vi "GUI.vi"() -> ()   [LabVIEW 2016]
uses:
  <vilib>/NI/Current Value Table/Type Defs/File Format.ctl
  <vilib>/NI/Current Value Table/Type Defs/Single Tag.ctl
  <vilib>/NI/Current Value Table/Type Defs/Data Types.ctl
  <vilib>/NI/Current Value Table/Type Defs/Tag Grouping set.ctl
  <vilib>/NI/Current Value Table/DataTypes/Boolean_Write.vi
  <vilib>/NI/Current Value Table/DataTypes/Boolean_Read.vi
  <vilib>/NI/Current Value Table/DataTypes/U16_Read.vi
  <vilib>/NI/Current Value Table/DataTypes/U16_Write.vi
  <vilib>/NI/Current Value Table/Type to Enum.vi
  <vilib>/NI/Current Value Table/DataTypes/Boolean_Type To Enum.vi
  <vilib>/NI/Current Value Table/DataTypes/U16_Type To Enum.vi
  MB_Master_Serial.lvclass
  C:/Users/PRANAV/Desktop/Modbus_Scada_Main/Modbus_Scada/MB_Master/MB_Master.lvclass
  MB_Master_TCP/MB_Master_TCP.lvclass
  <vilib>/NI/Current Value Table/FGVs/CVT Globals.vi
  <vilib>/NI/Current Value Table/FGVs/Tag Memory.vi
  <vilib>/NI/Current Value Table/Memory Block.vi
  <vilib>/NI/Current Value Table/DataTypes/Boolean_Memory Block.vi
  <vilib>/NI/Current Value Table/DataTypes/U16_Memory Block.vi
  MB_Master/MB_Master.lvclass
  <vilib>/NI/Current Value Table/Current Value Table.lvlib
  MB Master.lvlib
panel:
  in  "Type":enum16{"Serial", "TCP"}(ring) caption="Connection Type"
  out "Value_O2 3":u16
  out "Value_N2 3":u16
  out "Vel_Value 3":u16
  out "N2 Gas Pressure 1_Value 3":u16
  out "Temp_Min 4":u16
  out "Hum_Value  3":u16
  out "Value_O2 2":u16
  out "Value_N2 2":u16
  out "Vel_Value 2":u16
  out "N2 Gas Pressure 1_Value 2":u16
  out "Temp_Min 3":u16
  out "Hum_Value  2":u16
  out "Max_O2 2":u16
  out "Max_N2 2":u16
  out "Vel_Max 2":u16
  out "N2 Gas Pressure 1_Max 2":u16
  out "Temp_Max 2":u16
  out "Hum_Max 2":u16
  out "Min_O2 2":u16
  out "Min_N2 2":u16
  out "Vel_Min 2":u16
  out "N2 Gas Pressure 1_Min 2":u16
  out "Temp_Min 5":u16
  out "Hum_Min 2":u16
  out "Value_O2":u16
  out "Value_N2":u16
  out "Vel_Value":u16
  out "N2 Gas Pressure 1_Value":u16
  out "Temp_Min":u16
  out "Hum_Value":u16
  out "Spare AI-1_Value":u16
  out "Spare AI-2_Value":u16
  out "Max_O2":u16
  out "Max_N2":u16
  out "Vel_Max":u16
  out "N2 Gas Pressure 1_Max":u16
  out "Temp_Max":u16
  out "Hum_Max":u16
  out "Spare AI-1_Max":u16
  out "Spare AI-2_Max":u16
  out "Min_O2":u16
  out "Min_N2":u16
  out "Vel_Min":u16
  out "N2 Gas Pressure 1_Min":u16
  out "Temp_Min 2":u16
  out "Hum_Min":u16
  out "Spare AI-1_Min":u16
  out "Spare AI-2_Min":u16
  out "Value_8":bool
  out "Value_9":bool
  out "Value_10":bool
  out "Value_11":bool
  out "Value_12":bool
  out "Value_13":bool
  out "Value_14":bool
  out "Value_1":bool
  out "Value_2":bool
  out "Value_3":bool
  out "Value_4":bool
  out "Value_5":bool
  out "Value_6":bool
  out "Value_7":bool
  out "O.T. Entrance -Cap Proxy":bool
  out "Main Entrance E-stop PB":bool
  out "Doctors Entrance Door-2 Open Proxy FB":bool
  out "Main Entrance Door Open Inside PB":bool
  out "Main Entrance Door Open Proxy FB":bool
  out "O.T Entrance-Nose Mask Proxy":bool
  out "Doctors Entrance Door-1 Open PB":bool
  out "Doctors Entrance Door-1 Open Inside PB":bool
  out "Doctors Entrance Door-1 Open Proxy FB":bool
  out "Doctors Entrance-Nose Mask Proxy":bool
  out "Doctors Entrance-Cap Proxy":bool
  out "Doctors Entrance-Hand Sanitizer  Proxy":bool
  out "Doctors Entrance Door-2 Open Inside PB":bool
  out "Ist O.T.-Occupied Lamp Green":bool
  out "Ist O.T-AHU Start Coil":bool
  out "2nd O.T.:Scrubber Dispense Coil":bool
  out "2nd O.T.-Door Open Cmd":bool
  out "Spare DO-1":bool
  out "Spare DO-2":bool
  out "Spare DO-3":bool
  out "Spare DO-4":bool
  out "Spare DO-5":bool
  out "Spare DO-6":bool
  out "Doctor Entrance Door-1 Open Cmd":bool
  out "Doctor Entrance -Door-2 Open Cmd":bool
  out "Doctor Entrance -Hand Santizier Coil":bool
  out "Main Entrance-Door Open Cmd":bool
  out "OT Entrance-Door Open  Cmd":bool
  out "O.T Entrance-Hand Santiizier Coil":bool
  out "Ist O.T.- Door Open Cmd":bool
  out "Ist O.T-Occupied Lamp(Red)":bool
  out "Ist O.T-Inside Light":bool
  out "Ist O.T.-Scrubber Dispense Coil":bool
  out "error out":errorcluster
  in  "stop  5":bool
  in  "stop  4":bool
  in  "stop  3":bool
  in  "stop  2":bool
  in  "stop":bool
  # "DOORS &\n                    STATUS"
  # "Description"
  # "Status"
  # "Description"
  # "Status"
  # "Doctor Entrance Door-1 Open Cmd"
  # "Ist O.T.-Occupied Lamp Green"
  # "Doctor Entrance -Door-2 Open Cmd"
  # "Ist O.T-AHU Start Coil"
  # "Doctor Entrance -Hand Santizier Coil"
  # "2nd O.T.:Scrubber Dispense Coil"
  # "Main Entrance-Door Open Cmd"
  # "2nd O.T.-Door Open Cmd"
  # "OT Entrance-Door Open  Cmd"
  # "Spare DO-1"
  # "O.T Entrance-Hand Santiizier Coil"
  # "Spare DO-2"
  # "Ist O.T.- Door Open Cmd"
  # "Spare DO-3"
  # "Ist O.T-Occupied Lamp(Red)"
  # "Spare DO-4"
  # "Ist O.T-Inside Light"
  # "Spare DO-5"
  # "Ist O.T.-Scrubber Dispense Coil"
  # "Spare DO-6"
  # "DOORS FB AND SENSOR\n                                  STATUS"
  # "Description"
  # "Status"
  # "Description"
  # "Status"
  # "Doctors Entrance Door-1 Open PB"
  # "Doctors Entrance Door-2 Open Proxy FB"
  # "Doctors Entrance Door-1 Open Inside PB"
  # "Main Entrance E-stop PB"
  # "Doctors Entrance Door-1 Open Proxy FB"
  # "Main Entrance-Strecther Entry PB"
  # "Doctors Entrance-Nose Mask Proxy"
  # "Main Entrance Door Open Inside PB"
  # "Doctors Entrance-Cap Proxy"
  # "Main Entrance Door Open Proxy FB"
  # "Doctors Entrance-Hand Sanitizer  Proxy"
  # "O.T Entrance-Nose Mask Proxy"
  # "Doctors Entrance Door-2 Open Inside PB"
  # "O.T. Entrance -Cap Proxy"
  # "DOORS FB AND SENSOR\n                                  STATUS"
  # "Description"
  # "Status"
  # "Description"
  # "Status"
  # "OT Entrance-Hand Santizier Proxy"
  # "Spare DI-2"
  # "Spare DI-1"
  # "Ist O.T-AHU Run FB"
  # "OT Entrance-Door Inside Open PB"
  # "2nd O.T-Scrubber Proxy"
  # "OT Entrance-Door Open Proxy FB"
  # "2nd O.T-Door Inside Open PB"
  # "Ist O.T -Scrubber Proxy"
  # "2nd O.T-Door Open Proxy FB"
  # "Ist O.T-Door Inside Open PB"
  # "Ist O.T-E-Stop PB"
  # "Ist O.T-Door  Open Proxy FB"
  # "2nd O.T-E-Stop PB"
  # "O.T Parameters"
  # "Description"
  # "Min"
  # "Max"
  # "Value"
  # "Unit"
  # "O2 Gas Pressure"
  # "Bar"
  # "N2 Gas Pressure 1"
  # "Bar"
  # "Velocity"
  # "ft/m"
  # "N2 Gas Pressure 2"
  # "Bar"
  # "Room Temperature"
  # "Degree C"
  # "Relative Humidity"
  # "%"
  # "Spare AI 01"
  # "Spare AI 02"
  # "O.T Parameters S.P"
  # "Description"
  # "Very Low"
  # "Low"
  # "High"
  # "Very High"
  # "Unit"
  # "O2 Gas Pressure"
  # "Bar"
  # "N2 Gas Pressure 1"
  # "Bar"
  # "Velocity"
  # "ft/m"
  # "N2 Gas Pressure 2"
  # "Bar"
  # "Room Temperature"
  # "Degree C"
  # "Relative Humidity"
  # "%"
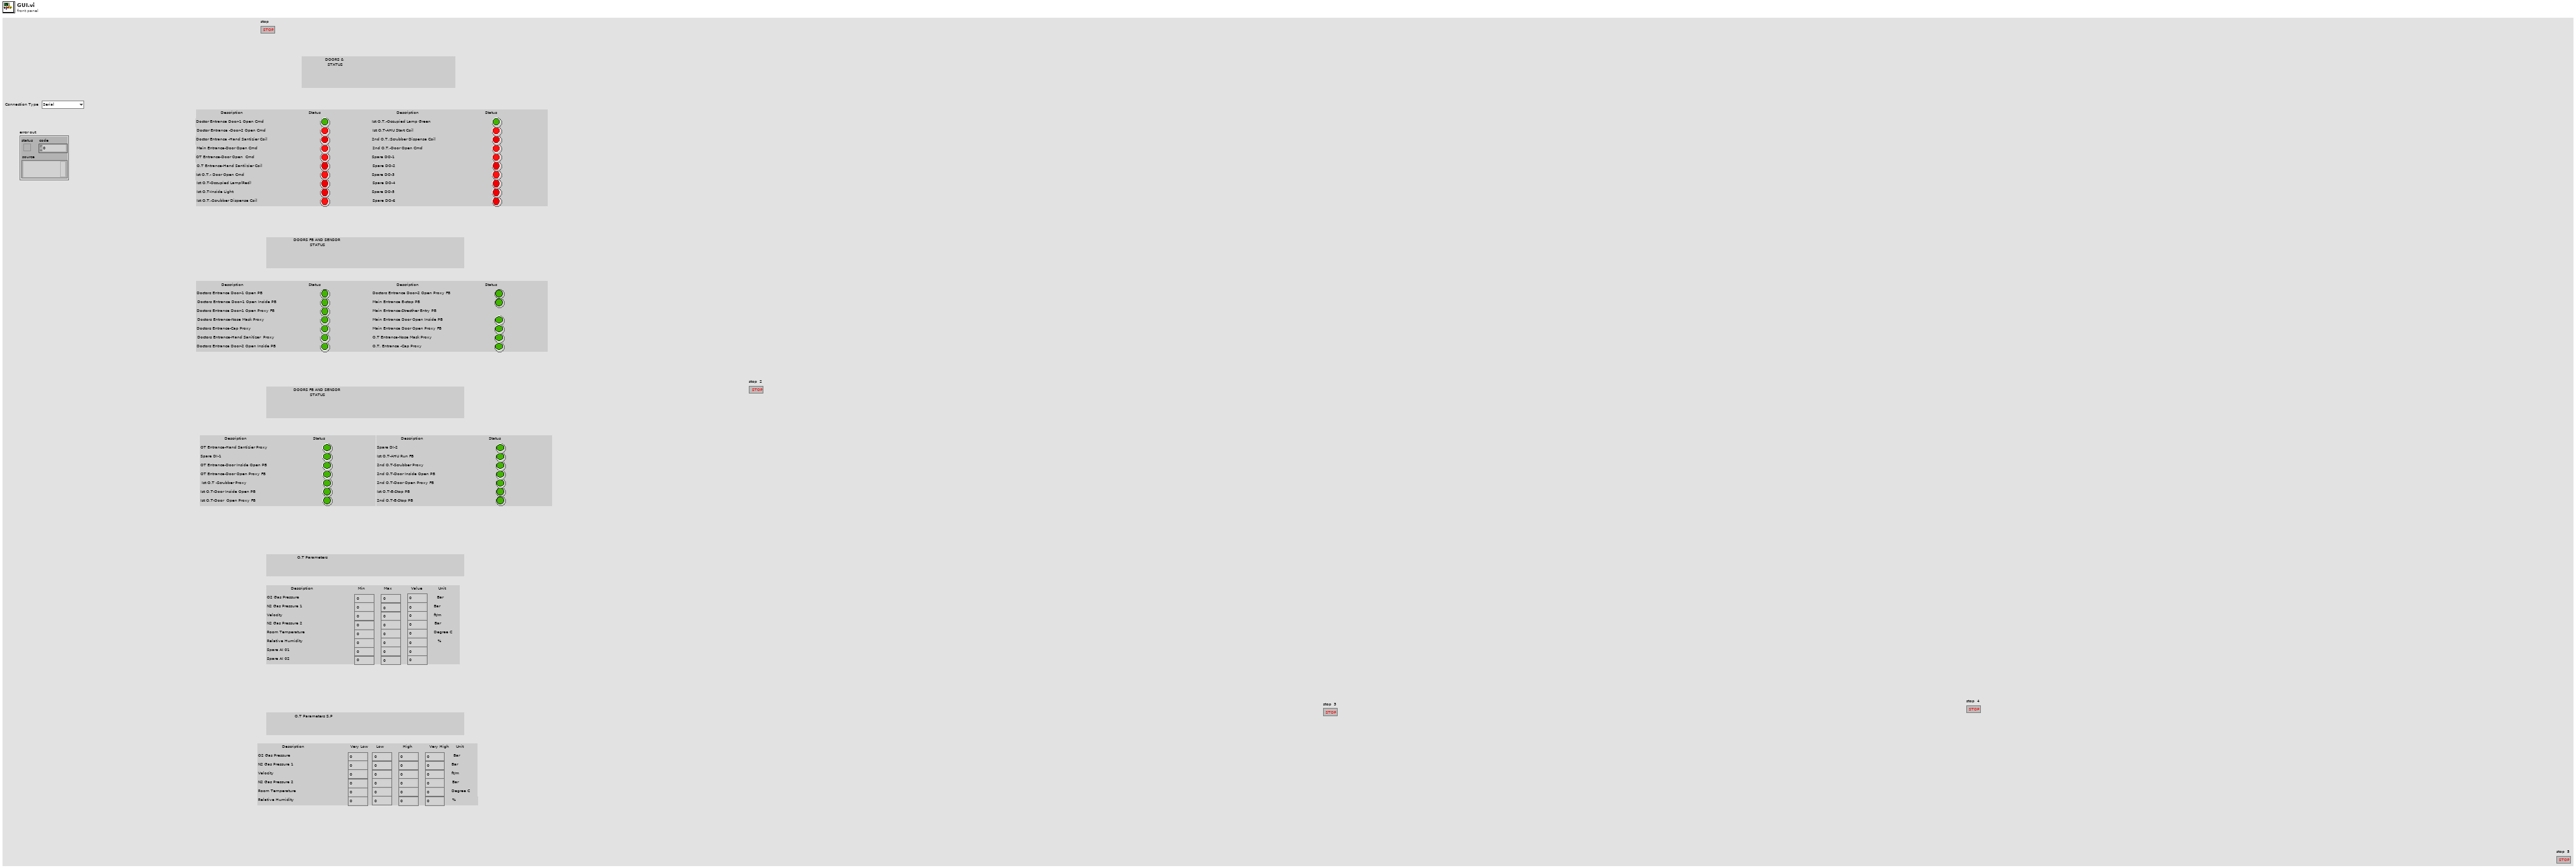
[diagram p1: front panel]
types:
  T1 = typedef "Current Value Table.lvlib/File Format.ctl" = cluster{"Tags":T2[], "Group Listings":T4[]}
  T2 = typedef "Current Value Table.lvlib/Single Tag.ctl" = cluster{"Data Type":T3, "Name":string, "Value":string, "Description":string}
  T3 = typedef "Current Value Table.lvlib/Data Types.ctl" = enum16{"Double", "Single", "I64", "I32", "I16", "I8", "U64", "U32", "U16", "U8", "String", "Boolean", "Array of U8", "Array of U16", "Array of U32", "Array of U64", "Array of I64", "Array of I32", "Array of I16", "Array of I8", "Array of Double", "Array of Single", "Array of Boolean", "Array of String"}
  T4 = typedef "Current Value Table.lvlib/Tag Grouping set.ctl" = cluster{"Group":string, "Tag Names":string[]}
  T5 = cluster{"baud rate (bps)":u32, "stop bits":u16, "parity":u16, "flow control":u16, "timeout":u32, "retries":i32}
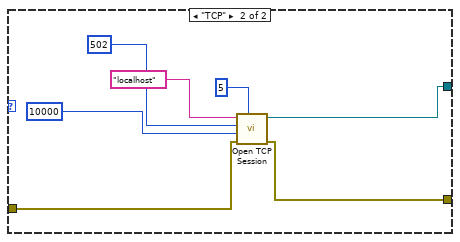
[diagram p2: hidden frame]
diagram:
  n1 = call <vilib>:"Create Tags.vi"("Clear Table? (F)"=FALSE, "CVT Tags to Create"=T1 {"Tags"=[{"Data Type"=enum."Boolean", "Name"="Doctor Entrance Door-1 Open Cmd", "Value"="", "Description"=""}, {"Data Type"=enum."Boolean", "Name"="Doctor Entrance -Door-2 Open Cmd", "Value"="", "Description"=""}, {"Data Type"=enum."Boolean", "Name"="Doctor Entrance -Hand Santizier Coil", "Value"="", "Description"=""}, {"Data Type"=enum."Boolean", "Name"="Main Entrance-Door Open Cmd", "Value"="", "Description"=""}, {"Data Type"=enum."Boolean", "Name"="OT Entrance-Door Open  Cmd", "Value"="", "Description"=""}, {"Data Type"=enum."Boolean", "Name"="O.T Entrance-Hand Santiizier Coil", "Value"="", "Description"=""}, {"Data Type"=enum."Boolean", "Name"="Ist O.T.- Door Open Cmd", "Value"="", "Description"=""}, {"Data Type"=enum."Boolean", "Name"="Ist O.T-Occupied Lamp(Red)", "Value"="", "Description"=""}, {"Data Type"=enum."Boolean", "Name"="Ist O.T-Inside Light", "Value"="", "Description"=""}, {"Data Type"=enum."Boolean", "Name"="Ist O.T.-Scrubber Dispense Coil", "Value"="", "Description"=""}, {"Data Type"=enum."Boolean", "Name"="Ist O.T.-Occupied Lamp Green", "Value"="", "Description"=""}, {"Data Type"=enum."Boolean", "Name"="Ist O.T-AHU Start Coil", "Value"="", "Description"=""}, {"Data Type"=enum."Boolean", "Name"="2nd O.T.:Scrubber Dispense Coil", "Value"="", "Description"=""}, {"Data Type"=enum."Boolean", "Name"="2nd O.T.-Door Open Cmd", "Value"="", "Description"=""}, {"Data Type"=enum."Boolean", "Name"="Spare DO-1", "Value"="", "Description"=""}, {"Data Type"=enum."Boolean", "Name"="Spare DO-2", "Value"="", "Description"=""}, {"Data Type"=enum."Boolean", "Name"="Spare DO-3", "Value"="", "Description"=""}, {"Data Type"=enum."Boolean", "Name"="Spare DO-4", "Value"="", "Description"=""}, {"Data Type"=enum."Boolean", "Name"="Spare DO-5", "Value"="", "Description"=""}, {"Data Type"=enum."Boolean", "Name"="Spare DO-6", "Value"="", "Description"=""}, {"Data Type"=enum."Boolean", "Name"="Doctors Entrance Door-1 Open PB ", "Value"="", "Description"=""}, {"Data Type"=enum."Boolean", "Name"="Doctors Entrance Door-1 Open Inside PB", "Value"="", "Description"=""}, {"Data Type"=enum."Boolean", "Name"="Doctors Entrance Door-1 Open Proxy FB", "Value"="", "Description"=""}, {"Data Type"=enum."Boolean", "Name"="Doctors Entrance-Nose Mask Proxy", "Value"="", "Description"=""}, {"Data Type"=enum."Boolean", "Name"="Doctors Entrance-Cap Proxy", "Value"="", "Description"=""}, {"Data Type"=enum."Boolean", "Name"="Doctors Entrance-Hand Sanitizer  Proxy", "Value"="", "Description"=""}, {"Data Type"=enum."Boolean", "Name"="Doctors Entrance Door-2 Open Inside PB", "Value"="", "Description"=""}, {"Data Type"=enum."Boolean", "Name"="Doctors Entrance Door-2 Open Proxy FB ", "Value"="", "Description"=""}, {"Data Type"=enum."Boolean", "Name"="Main Entrance E-stop PB", "Value"="", "Description"=""}, {"Data Type"=enum."Boolean", "Name"="Main Entrance-Strecther Entry PB ", "Value"="", "Description"=""}, {"Data Type"=enum."Boolean", "Name"="Main Entrance Door Open Inside PB", "Value"="", "Description"=""}, {"Data Type"=enum."Boolean", "Name"="Main Entrance Door Open Proxy FB", "Value"="", "Description"=""}, {"Data Type"=enum."Boolean", "Name"="O.T Entrance-Nose Mask Proxy ", "Value"="", "Description"=""}, {"Data Type"=enum."Boolean", "Name"="O.T. Entrance -Cap Proxy", "Value"="", "Description"=""}, {"Data Type"=enum."Boolean", "Name"="OT Entrance-Hand Santizier Proxy", "Value"="", "Description"=""}, {"Data Type"=enum."Boolean", "Name"="Spare DI-1", "Value"="", "Description"=""}, {"Data Type"=enum."Boolean", "Name"="OT Entrance-Door Inside Open PB ", "Value"="", "Description"=""}, {"Data Type"=enum."Boolean", "Name"="OT Entrance-Door Open Proxy FB ", "Value"="", "Description"=""}, {"Data Type"=enum."Boolean", "Name"="Ist O.T -Scrubber Proxy", "Value"="", "Description"=""}, {"Data Type"=enum."Boolean", "Name"="Ist O.T-Door Inside Open PB", "Value"="", "Description"=""}, {"Data Type"=enum."Boolean", "Name"="Ist O.T-Door  Open Proxy FB ", "Value"="", "Description"=""}, {"Data Type"=enum."Boolean", "Name"="Spare DI-2", "Value"="", "Description"=""}, {"Data Type"=enum."Boolean", "Name"="Ist O.T-AHU Run FB", "Value"="", "Description"=""}, {"Data Type"=enum."Boolean", "Name"="2nd O.T-Scrubber Proxy", "Value"="", "Description"=""}, {"Data Type"=enum."Boolean", "Name"="2nd O.T-Door Inside Open PB", "Value"="", "Description"=""}, {"Data Type"=enum."Boolean", "Name"="2nd O.T-Door Open Proxy FB ", "Value"="", "Description"=""}, {"Data Type"=enum."Boolean", "Name"="Ist O.T-E-Stop PB", "Value"="", "Description"=""}, {"Data Type"=enum."Boolean", "Name"="2nd O.T-E-Stop PB ", "Value"="", "Description"=""}, {"Data Type"=enum."U16", "Name"="O2 Gas Pressure_Min", "Value"="", "Description"=""}, {"Data Type"=enum."Double", "Name"="O2 Gas Pressure", "Value"="", "Description"=""}, {"Data Type"=enum."U16", "Name"="O2 Gas Pressure _Value", "Value"="", "Description"=""}, {"Data Type"=enum."U16", "Name"="O2 Gas Pressure_Max", "Value"="", "Description"=""}, {"Data Type"=enum."U16", "Name"="N2 Gas Pressure_Min", "Value"="", "Description"=""}, {"Data Type"=enum."U16", "Name"="N2 Gas Pressure_Max", "Value"="", "Description"=""}, {"Data Type"=enum."U16", "Name"="N2 Gas Pressure_Value", "Value"="", "Description"=""}, {"Data Type"=enum."U16", "Name"="Velocity_Min", "Value"="", "Description"=""}, {"Data Type"=enum."U16", "Name"="Velocity_Max", "Value"="", "Description"=""}, {"Data Type"=enum."U16", "Name"="Velocity_Value", "Value"="", "Description"=""}, {"Data Type"=enum."U16", "Name"="N2 Gas Pressure 1_Min", "Value"="", "Description"=""}, {"Data Type"=enum."U16", "Name"="N2 Gas Pressure 1 _Max", "Value"="", "Description"=""}, {"Data Type"=enum."U16", "Name"="N2 Gas Pressure 1_Value", "Value"="", "Description"=""}, {"Data Type"=enum."U16", "Name"="Temp_Min", "Value"="", "Description"=""}, {"Data Type"=enum."U16", "Name"="Temp_Max", "Value"="", "Description"=""}, {"Data Type"=enum."U16", "Name"="Temp_Value", "Value"="", "Description"=""}, {"Data Type"=enum."U16", "Name"="Hum_Min", "Value"="", "Description"=""}, {"Data Type"=enum."U16", "Name"="Hum_Max", "Value"="", "Description"=""}, {"Data Type"=enum."U16", "Name"="Hum_Value", "Value"="", "Description"=""}, {"Data Type"=enum."U16", "Name"="Spare AI-1_Min", "Value"="", "Description"=""}, {"Data Type"=enum."U16", "Name"="Spare AI-1_Max", "Value"="", "Description"=""}, {"Data Type"=enum."U16", "Name"="Spare AI-1_Value", "Value"="", "Description"=""}, {"Data Type"=enum."U16", "Name"="Spare AI-2_Min", "Value"="", "Description"=""}, {"Data Type"=enum."U16", "Name"="Spare AI-2_Max", "Value"="", "Description"=""}, {"Data Type"=enum."U16", "Name"="Spare AI-2_Value", "Value"="", "Description"=""}, {"Data Type"=enum."Boolean", "Name"="Value_1", "Value"="", "Description"=""}, {"Data Type"=enum."Boolean", "Name"="Value_2", "Value"="", "Description"=""}, {"Data Type"=enum."Boolean", "Name"="Value_3", "Value"="", "Description"=""}, {"Data Type"=enum."Boolean", "Name"="Value_4", "Value"="", "Description"=""}, {"Data Type"=enum."Boolean", "Name"="Value_5", "Value"="", "Description"=""}, {"Data Type"=enum."Boolean", "Name"="Value_6", "Value"="", "Description"=""}, {"Data Type"=enum."Boolean", "Name"="Value_7", "Value"="", "Description"=""}, {"Data Type"=enum."Boolean", "Name"="Value_8", "Value"="", "Description"=""}, {"Data Type"=enum."Boolean", "Name"="Value_9", "Value"="", "Description"=""}, {"Data Type"=enum."Boolean", "Name"="Value_10", "Value"="", "Description"=""}, {"Data Type"=enum."Boolean", "Name"="Value_11", "Value"="", "Description"=""}, {"Data Type"=enum."Boolean", "Name"="Value_12", "Value"="", "Description"=""}, {"Data Type"=enum."Boolean", "Name"="Value_13", "Value"="", "Description"=""}, {"Data Type"=enum."Boolean", "Name"="Value_14", "Value"="", "Description"=""}, {"Data Type"=enum."U16", "Name"="O2_L1", "Value"="", "Description"=""}, {"Data Type"=enum."U16", "Name"="O2_L2", "Value"="", "Description"=""}, {"Data Type"=enum."U16", "Name"="O2_H1", "Value"="", "Description"=""}, {"Data Type"=enum."U16", "Name"="O2_H2", "Value"="", "Description"=""}, {"Data Type"=enum."U16", "Name"="N21_L1", "Value"="", "Description"=""}, {"Data Type"=enum."U16", "Name"="N21_L2", "Value"="", "Description"=""}, {"Data Type"=enum."U16", "Name"="N21_H1", "Value"="", "Description"=""}, {"Data Type"=enum."U16", "Name"="N21_H2", "Value"="", "Description"=""}, {"Data Type"=enum."U16", "Name"="Vel_L1", "Value"="", "Description"=""}, {"Data Type"=enum."U16", "Name"="Vel_L2", "Value"="", "Description"=""}, {"Data Type"=enum."U16", "Name"="Vel_H1", "Value"="", "Description"=""}, {"Data Type"=enum."U16", "Name"="Vel_H2", "Value"="", "Description"=""}, {"Data Type"=enum."U16", "Name"="N22_L1", "Value"="", "Description"=""}, {"Data Type"=enum."U16", "Name"="N22_L2", "Value"="", "Description"=""}, {"Data Type"=enum."U16", "Name"="N22_H1", "Value"="", "Description"=""}, {"Data Type"=enum."U16", "Name"="N22_H2", "Value"="", "Description"=""}, {"Data Type"=enum."U16", "Name"="Temp_L1", "Value"="", "Description"=""}, {"Data Type"=enum."U16", "Name"="Temp_L2", "Value"="", "Description"=""}, {"Data Type"=enum."U16", "Name"="Temp_H1", "Value"="", "Description"=""}, {"Data Type"=enum."U16", "Name"="Temp_H2", "Value"="", "Description"=""}, {"Data Type"=enum."U16", "Name"="RH_L1", "Value"="", "Description"=""}, {"Data Type"=enum."U16", "Name"="RH_L2", "Value"="", "Description"=""}, {"Data Type"=enum."U16", "Name"="RH_H1", "Value"="", "Description"=""}, {"Data Type"=enum."U16", "Name"="RH_H2", "Value"="", "Description"=""}], "Group Listings"=[]}) -> ("error out"=w4:errorcluster)  [unwired: 9 in]
  n2 = case shown="\"Serial\", Default" "Type" {
    tunnel: [w14 w19] -> w2
    tunnel: [w13 w20] -> w3
    tunnel: w4 -> [w10 w17]
    frame "Serial", Default {
      n3 = call "Open Serial Session.vi"("Mode (RTU)"=enum16{"RTU", "ASCII"}."RTU", "Error in"=w10, "Slave ID"=u8 5, "Serial Config"=T5 {"baud rate (bps)"=19200, "stop bits"=10, "parity"=0, "flow control"=0, "timeout"=1000, "retries"=1}, "VISA Resource"=refnum<visa-resource-name> "COM9") -> ("Error out"=w14:errorcluster, "MB_Serial session"=w13:refnum<class "MB_Master_Serial.lvclass">)  [unwired: 5 in]
    }
    frame "TCP" {
      n4 = call "Open TCP Session.vi"("Slave ID (255)"=u8 5, "error in (no error)"=w17, "Timeout (10000)"=10000, "Port (502)"=u16 502, "IP Address"="localhost") -> ("error out"=w19:errorcluster, "MB_TCP session"=w20:refnum<class "MB_Master_TCP.lvclass">)  [unwired: 5 in]
    }
  }
  n5 = while {
    shift-right: [w39] -> w7
    shift-left: w3 -> [w40]
    shift-right: [w38] -> w6
    shift-left: w2 -> [w41]
    stop <- w24 stop-if-true
    n6 = flat-sequence {
      tunnel: w41 -> [w43]
      tunnel: w40 -> [w44]
      tunnel: [w168] -> w37
      tunnel: [w50] -> w36
      tunnel: [w46] -> w35
      tunnel: [w42] -> w34
      tunnel: w37 -> [_]
      tunnel: w36 -> [w177]
      tunnel: w35 -> [_]
      tunnel: w34 -> [w178]
      tunnel: [w247] -> w33
      tunnel: [w173] -> w32
      tunnel: [w172] -> w31
      tunnel: w33 -> [_]
      tunnel: w32 -> [w265]
      tunnel: w31 -> [w266]
      tunnel: [w400] -> w30
      tunnel: [w261] -> w29
      tunnel: [w262] -> w28
      tunnel: w30 -> [_]
      tunnel: w29 -> [w421]
      tunnel: w28 -> [w424]
      tunnel: [w420] -> w27
      tunnel: [w422] -> w26
      tunnel: [w504] -> w25
      tunnel: [w515] -> w39
      tunnel: [w516] -> w38
      tunnel: w27 -> [w517]
      tunnel: w26 -> [w513]
      tunnel: w25 -> [_]
      tunnel: [w636] -> w24
      frame #0 {
        w55 = "Spare DO-6" ("Tag Name")
        w62 = "Spare DO-5" ("Tag Name")
        w66 = "Spare DO-4" ("Tag Name")
        w70 = "Spare DO-3" ("Tag Name")
        w76 = "Spare DO-2" ("Tag Name")
        w49 = "Spare DO-1" ("Tag Name")
        w89 = "2nd O.T.-Door Open Cmd" ("Tag Name")
        w94 = "2nd O.T.:Scrubber Dispense Coil" ("Tag Name")
        w101 = "Ist O.T-AHU Start Coil" ("Tag Name")
        w104 = "Ist O.T.-Occupied Lamp Green" ("Tag Name")
        w113 = "Ist O.T.-Scrubber Dispense Coil" ("Tag Name")
        w117 = "Ist O.T-Inside Light" ("Tag Name")
        w125 = "Ist O.T-Occupied Lamp(Red)" ("Tag Name")
        w130 = "Ist O.T.- Door Open Cmd" ("Tag Name")
        w135 = "O.T Entrance-Hand Santiizier Coil" ("Tag Name")
        w153 = "OT Entrance-Door Open  Cmd" ("Tag Name")
        w156 = "Main Entrance-Door Open Cmd" ("Tag Name")
        w159 = "Doctor Entrance -Hand Santizier Coil" ("Tag Name")
        w165 = "Doctor Entrance -Door-2 Open Cmd" ("Tag Name")
        w171 = "Doctor Entrance Door-1 Open Cmd" ("Tag Name")
        n7 = call "Read Coils.vi"("error in (no error)"=w43, "quantity"=u16 22, "starting address"=u16 0, "MB session in"=w44) -> ("error out"=w45:errorcluster, "Coils"=w46:bool[], "MB session out"=w42:refnum<class "MB_Master.lvclass">)  [unwired: 5 in]
        n8 = Index Array(array=w46, index #1=0 ("index"), index #2=1 ("index"), index #3=2 ("index"), index #4=3 ("index"), index #5=4 ("index"), index #6=5 ("index"), index #7=6 ("index"), index #8=7 ("index"), index #9=8 ("index"), index #10=9 ("index"), index #11=10 ("index"), index #12=11 ("index"), index #13=12 ("index"), index #14=13 ("index"), index #15=14 ("index"), index #16=15 ("index"), index #17=16 ("index"), index #18=17 ("index"), index #19=18 ("index"), index #20=19 ("index")) -> (element #1=w148:bool, element #2=w146:bool, element #3=w144:bool, element #4=w142:bool, element #5=w140:bool, element #6=w138:bool, element #7=w132:bool, element #8=w126:bool, element #9=w120:bool, element #10=w114:bool, element #11=w108:bool, element #12=w102:bool, element #13=w96:bool, element #14=w90:bool, element #15=w83:bool, element #16=w78:bool, element #17=w73:bool, element #18=w67:bool, element #19=w63:bool, element #20=w54:bool)
        n9 = call-poly <vilib>:"Write.vi"("error in (no error)"=w45, "Value"=w148, "Tag Name"=w171) -> ("error out"=w164:errorcluster)  [unwired: 8 in]
        n10 = call-poly <vilib>:"Write.vi"("error in (no error)"=w164, "Value"=w146, "Tag Name"=w165) -> ("error out"=w161:errorcluster)  [unwired: 8 in]
        n11 = call-poly <vilib>:"Write.vi"("error in (no error)"=w161, "Value"=w144, "Tag Name"=w159) -> ("error out"=w157:errorcluster)  [unwired: 8 in]
        n12 = call-poly <vilib>:"Write.vi"("error in (no error)"=w157, "Value"=w142, "Tag Name"=w156) -> ("error out"=w150:errorcluster)  [unwired: 8 in]
        n13 = call-poly <vilib>:"Write.vi"("error in (no error)"=w150, "Value"=w140, "Tag Name"=w153) -> ("error out"=w137:errorcluster)  [unwired: 8 in]
        n14 = call-poly <vilib>:"Write.vi"("error in (no error)"=w137, "Value"=w138, "Tag Name"=w135) -> ("error out"=w131:errorcluster)  [unwired: 8 in]
        n15 = call-poly <vilib>:"Write.vi"("error in (no error)"=w131, "Value"=w132, "Tag Name"=w130) -> ("error out"=w124:errorcluster)  [unwired: 8 in]
        n16 = call-poly <vilib>:"Write.vi"("error in (no error)"=w124, "Value"=w126, "Tag Name"=w125) -> ("error out"=w119:errorcluster)  [unwired: 8 in]
        n17 = call-poly <vilib>:"Write.vi"("error in (no error)"=w119, "Value"=w120, "Tag Name"=w117) -> ("error out"=w112:errorcluster)  [unwired: 8 in]
        n18 = call-poly <vilib>:"Write.vi"("error in (no error)"=w112, "Value"=w114, "Tag Name"=w113) -> ("error out"=w105:errorcluster)  [unwired: 8 in]
        n19 = call-poly <vilib>:"Write.vi"("error in (no error)"=w105, "Value"=w108, "Tag Name"=w104) -> ("error out"=w100:errorcluster)  [unwired: 8 in]
        n20 = call-poly <vilib>:"Write.vi"("error in (no error)"=w100, "Value"=w102, "Tag Name"=w101) -> ("error out"=w95:errorcluster)  [unwired: 8 in]
        n21 = call-poly <vilib>:"Write.vi"("error in (no error)"=w95, "Value"=w96, "Tag Name"=w94) -> ("error out"=w88:errorcluster)  [unwired: 8 in]
        n22 = call-poly <vilib>:"Write.vi"("error in (no error)"=w88, "Value"=w90, "Tag Name"=w89) -> ("error out"=w85:errorcluster)  [unwired: 8 in]
        n23 = call-poly <vilib>:"Write.vi"("error in (no error)"=w85, "Value"=w83, "Tag Name"=w49) -> ("error out"=w80:errorcluster)  [unwired: 8 in]
        n24 = call-poly <vilib>:"Write.vi"("error in (no error)"=w80, "Value"=w78, "Tag Name"=w76) -> ("error out"=w72:errorcluster)  [unwired: 8 in]
        n25 = call-poly <vilib>:"Write.vi"("error in (no error)"=w72, "Value"=w73, "Tag Name"=w70) -> ("error out"=w60:errorcluster)  [unwired: 8 in]
        n26 = call-poly <vilib>:"Write.vi"("error in (no error)"=w60, "Value"=w67, "Tag Name"=w66) -> ("error out"=w61:errorcluster)  [unwired: 8 in]
        n27 = call-poly <vilib>:"Write.vi"("error in (no error)"=w61, "Value"=w63, "Tag Name"=w62) -> ("error out"=w53:errorcluster)  [unwired: 8 in]
        n28 = call-poly <vilib>:"Write.vi"("error in (no error)"=w53, "Value"=w54, "Tag Name"=w55) -> ()  [unwired: 8 in, 1 out]
        n29 = call-poly <vilib>:"Read.vi"("error in (no error)"=w164, "Tag Name"=w171) -> ("error out"=w163:errorcluster, "Value"=→"Doctor Entrance Door-1 Open Cmd":bool)  [unwired: 8 in]
        n30 = call-poly <vilib>:"Read.vi"("error in (no error)"=w163, "Tag Name"=w165) -> ("error out"=w160:errorcluster, "Value"=→"Doctor Entrance -Door-2 Open Cmd":bool)  [unwired: 8 in]
        n31 = call-poly <vilib>:"Read.vi"("error in (no error)"=w160, "Tag Name"=w159) -> ("error out"=w155:errorcluster, "Value"=→"Doctor Entrance -Hand Santizier Coil":bool)  [unwired: 8 in]
        n32 = Wait (ms)(milliseconds to wait=u32 500) -> ()  [unwired: 1 out]
        n33 = call-poly <vilib>:"Read.vi"("error in (no error)"=w155, "Tag Name"=w156) -> ("error out"=w152:errorcluster, "Value"=→"Main Entrance-Door Open Cmd":bool)  [unwired: 8 in]
        n34 = call-poly <vilib>:"Read.vi"("error in (no error)"=w152, "Tag Name"=w153) -> ("error out"=w136:errorcluster, "Value"=→"OT Entrance-Door Open  Cmd":bool)  [unwired: 8 in]
        n35 = call-poly <vilib>:"Read.vi"("error in (no error)"=w136, "Tag Name"=w135) -> ("error out"=w129:errorcluster, "Value"=→"O.T Entrance-Hand Santiizier Coil":bool)  [unwired: 8 in]
        n36 = call-poly <vilib>:"Read.vi"("error in (no error)"=w129, "Tag Name"=w130) -> ("error out"=w123:errorcluster, "Value"=→"Ist O.T.- Door Open Cmd":bool)  [unwired: 8 in]
        n37 = call-poly <vilib>:"Read.vi"("error in (no error)"=w123, "Tag Name"=w125) -> ("error out"=w118:errorcluster, "Value"=→"Ist O.T-Occupied Lamp(Red)":bool)  [unwired: 8 in]
        n38 = call-poly <vilib>:"Read.vi"("error in (no error)"=w118, "Tag Name"=w117) -> ("error out"=w111:errorcluster, "Value"=→"Ist O.T-Inside Light":bool)  [unwired: 8 in]
        n39 = call-poly <vilib>:"Read.vi"("error in (no error)"=w111, "Tag Name"=w113) -> ("error out"=w106:errorcluster, "Value"=→"Ist O.T.-Scrubber Dispense Coil":bool)  [unwired: 8 in]
        n40 = call-poly <vilib>:"Read.vi"("error in (no error)"=w106, "Tag Name"=w104) -> ("error out"=w99:errorcluster, "Value"=→"Ist O.T.-Occupied Lamp Green":bool)  [unwired: 8 in]
        n41 = call-poly <vilib>:"Read.vi"("error in (no error)"=w99, "Tag Name"=w101) -> ("error out"=w93:errorcluster, "Value"=→"Ist O.T-AHU Start Coil":bool)  [unwired: 8 in]
        n42 = call-poly <vilib>:"Read.vi"("error in (no error)"=w93, "Tag Name"=w94) -> ("error out"=w87:errorcluster, "Value"=→"2nd O.T.:Scrubber Dispense Coil":bool)  [unwired: 8 in]
        n43 = call-poly <vilib>:"Read.vi"("error in (no error)"=w87, "Tag Name"=w89) -> ("error out"=w82:errorcluster, "Value"=→"2nd O.T.-Door Open Cmd":bool)  [unwired: 8 in]
        n44 = call-poly <vilib>:"Read.vi"("error in (no error)"=w82, "Tag Name"=w49) -> ("error out"=w77:errorcluster, "Value"=→"Spare DO-1":bool)  [unwired: 8 in]
        n45 = call-poly <vilib>:"Read.vi"("error in (no error)"=w77, "Tag Name"=w76) -> ("error out"=w71:errorcluster, "Value"=→"Spare DO-2":bool)  [unwired: 8 in]
        n46 = call-poly <vilib>:"Read.vi"("error in (no error)"=w71, "Tag Name"=w70) -> ("error out"=w59:errorcluster, "Value"=→"Spare DO-3":bool)  [unwired: 8 in]
        n47 = call-poly <vilib>:"Read.vi"("error in (no error)"=w59, "Tag Name"=w66) -> ("error out"=w58:errorcluster, "Value"=→"Spare DO-4":bool)  [unwired: 8 in]
        n48 = call-poly <vilib>:"Read.vi"("error in (no error)"=w58, "Tag Name"=w62) -> ("error out"=w52:errorcluster, "Value"=→"Spare DO-5":bool)  [unwired: 8 in]
        n49 = call-poly <vilib>:"Read.vi"("error in (no error)"=w52, "Tag Name"=w55) -> ("error out"=w50:errorcluster, "Value"=→"Spare DO-6":bool)  [unwired: 8 in]
        n50 = Unbundle By Name(w50) -> ("status"=w169:bool)
        n51 = Or(x=w169, y="stop") -> (x .or. y?=w168:bool)
      }
      frame #1 {
        w185 = "O.T Entrance-Nose Mask Proxy " ("Tag Name")
        w190 = "Main Entrance Door Open Proxy FB" ("Tag Name")
        w195 = "Main Entrance Door Open Inside PB" ("Tag Name")
        w201 = "Doctors Entrance Door-2 Open Proxy FB " ("Tag Name")
        w207 = "Main Entrance E-stop PB" ("Tag Name")
        (unwired) FALSE ("Value")
        w213 = "O.T. Entrance -Cap Proxy" ("Tag Name")
        w221 = "Doctors Entrance Door-2 Open Inside PB" ("Tag Name")
        w224 = "Doctors Entrance-Hand Sanitizer  Proxy" ("Tag Name")
        w231 = "Doctors Entrance-Cap Proxy" ("Tag Name")
        w238 = "Doctors Entrance-Nose Mask Proxy" ("Tag Name")
        w244 = "Doctors Entrance Door-1 Open Proxy FB" ("Tag Name")
        w251 = "Doctors Entrance Door-1 Open Inside PB" ("Tag Name")
        w256 = "Doctors Entrance Door-1 Open PB " ("Tag Name")
        n52 = call "Read Discrete Inputs.vi"("error in (no error)"=w177, "quantity"=u16 16 ("Quantity"), "starting address"=u16 0 ("Starting Address"), "MB session in"=w178) -> ("error out"=w173:errorcluster, "Inputs"=w174:bool[], "MB session out"=w172:refnum<class "MB_Master.lvclass">)  [unwired: 5 in]
        n53 = Index Array(array=w174, index #1=0 ("index"), index #2=1 ("index"), index #3=2 ("index"), index #4=3 ("index"), index #5=4 ("index"), index #6=5 ("index"), index #7=6 ("index"), index #8=8 ("index"), index #9=9 ("index"), index #10=10 ("index"), index #11=11 ("index"), index #12=12 ("index"), index #13=13 ("index"), index #14=14 ("index")) -> (element #1=w259:bool, element #2=w252:bool, element #3=w245:bool, element #4=w239:bool, element #5=w233:bool, element #6=w225:bool, element #7=w219:bool, element #8=w215:bool, element #9=w209:bool, element #10=w202:bool, element #12=w196:bool, element #13=w192:bool, element #14=w186:bool)  [unwired: 1 out]
        n54 = call-poly <vilib>:"Write.vi"("Value"=w259, "Tag Name"=w256) -> ("error out"=w258:errorcluster)  [unwired: 9 in]
        n55 = call-poly <vilib>:"Write.vi"("error in (no error)"=w258, "Value"=w252, "Tag Name"=w251) -> ("error out"=w242:errorcluster)  [unwired: 8 in]
        n56 = call-poly <vilib>:"Write.vi"("error in (no error)"=w242, "Value"=w245, "Tag Name"=w244) -> ("error out"=w237:errorcluster)  [unwired: 8 in]
        n57 = call-poly <vilib>:"Write.vi"("error in (no error)"=w237, "Value"=w239, "Tag Name"=w238) -> ("error out"=w232:errorcluster)  [unwired: 8 in]
        n58 = call-poly <vilib>:"Write.vi"("error in (no error)"=w232, "Value"=w233, "Tag Name"=w231) -> ("error out"=w228:errorcluster)  [unwired: 8 in]
        n59 = call-poly <vilib>:"Write.vi"("error in (no error)"=w228, "Value"=w225, "Tag Name"=w224) -> ("error out"=w220:errorcluster)  [unwired: 8 in]
        n60 = call-poly <vilib>:"Write.vi"("error in (no error)"=w220, "Value"=w219, "Tag Name"=w221) -> ("error out"=w214:errorcluster)  [unwired: 8 in]
        n61 = call-poly <vilib>:"Write.vi"("error in (no error)"=w214, "Value"=w215, "Tag Name"=w213) -> ("error out"=w208:errorcluster)  [unwired: 8 in]
        n62 = call-poly <vilib>:"Write.vi"("error in (no error)"=w208, "Value"=w209, "Tag Name"=w207) -> ("error out"=w203:errorcluster)  [unwired: 8 in]
        n63 = call-poly <vilib>:"Write.vi"("error in (no error)"=w203, "Value"=w202, "Tag Name"=w201) -> ("error out"=w180:errorcluster)  [unwired: 8 in]
        n64 = call-poly <vilib>:"Write.vi"("error in (no error)"=w180, "Value"=w196, "Tag Name"=w195) -> ("error out"=w191:errorcluster)  [unwired: 8 in]
        n65 = call-poly <vilib>:"Write.vi"("error in (no error)"=w191, "Value"=w192, "Tag Name"=w190) -> ("error out"=w184:errorcluster)  [unwired: 8 in]
        n66 = call-poly <vilib>:"Write.vi"("error in (no error)"=w184, "Value"=w186, "Tag Name"=w185) -> ()  [unwired: 8 in, 1 out]
        n67 = call-poly <vilib>:"Read.vi"("error in (no error)"=w258, "Tag Name"=w256) -> ("error out"=w257:errorcluster, "Value"=→"Doctors Entrance Door-1 Open PB":bool)  [unwired: 8 in]
        n68 = call-poly <vilib>:"Read.vi"("error in (no error)"=w257, "Tag Name"=w251) -> ("error out"=w243:errorcluster, "Value"=→"Doctors Entrance Door-1 Open Inside PB":bool)  [unwired: 8 in]
        n69 = call-poly <vilib>:"Read.vi"("error in (no error)"=w243, "Tag Name"=w244) -> ("error out"=w236:errorcluster, "Value"=→"Doctors Entrance Door-1 Open Proxy FB":bool)  [unwired: 8 in]
        n70 = call-poly <vilib>:"Read.vi"("error in (no error)"=w236, "Tag Name"=w238) -> ("error out"=w230:errorcluster, "Value"=→"Doctors Entrance-Nose Mask Proxy":bool)  [unwired: 8 in]
        n71 = call-poly <vilib>:"Read.vi"("error in (no error)"=w230, "Tag Name"=w231) -> ("error out"=w227:errorcluster, "Value"=→"Doctors Entrance-Cap Proxy":bool)  [unwired: 8 in]
        n72 = call-poly <vilib>:"Read.vi"("error in (no error)"=w227, "Tag Name"=w224) -> ("error out"=w217:errorcluster, "Value"=→"Doctors Entrance-Hand Sanitizer  Proxy":bool)  [unwired: 8 in]
        n73 = call-poly <vilib>:"Read.vi"("error in (no error)"=w217, "Tag Name"=w221) -> ("error out"=w212:errorcluster, "Value"=→"Doctors Entrance Door-2 Open Inside PB":bool)  [unwired: 8 in]
        n74 = call-poly <vilib>:"Read.vi"("error in (no error)"=w212, "Tag Name"=w213) -> ("error out"=w206:errorcluster, "Value"=→"O.T. Entrance -Cap Proxy":bool)  [unwired: 8 in]
        n75 = call-poly <vilib>:"Read.vi"("error in (no error)"=w206, "Tag Name"=w207) -> ("error out"=w200:errorcluster, "Value"=→"Main Entrance E-stop PB":bool)  [unwired: 8 in]
        n76 = call-poly <vilib>:"Read.vi"("error in (no error)"=w200, "Tag Name"=w201) -> ("error out"=w179:errorcluster, "Value"=→"Doctors Entrance Door-2 Open Proxy FB":bool)  [unwired: 8 in]
        n77 = call-poly <vilib>:"Read.vi"("error in (no error)"=w179, "Tag Name"=w195) -> ("error out"=w189:errorcluster, "Value"=→"Main Entrance Door Open Inside PB":bool)  [unwired: 8 in]
        n78 = call-poly <vilib>:"Read.vi"("error in (no error)"=w189, "Tag Name"=w190) -> ("error out"=w183:errorcluster, "Value"=→"Main Entrance Door Open Proxy FB":bool)  [unwired: 8 in]
        n79 = call-poly <vilib>:"Read.vi"("error in (no error)"=w183, "Tag Name"=w185) -> ("error out"=w182:errorcluster, "Value"=→"O.T Entrance-Nose Mask Proxy":bool)  [unwired: 8 in]
        n80 = Unbundle By Name(w182) -> ("status"=w248:bool)
        n81 = Or(x=w248, y="stop  2") -> (x .or. y?=w247:bool)
      }
      frame #2 {
        w274 = "Spare AI-2_Min" ("Tag Name")
        w275 = "Spare AI-2_Value" ("Tag Name")
        w276 = "Spare AI-2_Max" ("Tag Name")
        w293 = "Spare AI-1_Value" ("Tag Name")
        w294 = "Spare AI-1_Max" ("Tag Name")
        w296 = "Spare AI-1_Min" ("Tag Name")
        w310 = "Hum_Value" ("Tag Name")
        w311 = "Hum_Max" ("Tag Name")
        w312 = "Hum_Min" ("Tag Name")
        w330 = "Temp_Value" ("Tag Name")
        w329 = "Temp_Max" ("Tag Name")
        w327 = "Temp_Min" ("Tag Name")
        w343 = "N2 Gas Pressure 1_Value" ("Tag Name")
        w348 = "N2 Gas Pressure 1 _Max" ("Tag Name")
        w349 = "N2 Gas Pressure 1_Min" ("Tag Name")
        w363 = "Velocity_Value" ("Tag Name")
        w365 = "Velocity_Max" ("Tag Name")
        w368 = "Velocity_Min" ("Tag Name")
        w383 = "N2 Gas Pressure_Value" ("Tag Name")
        w388 = "N2 Gas Pressure_Max" ("Tag Name")
        w392 = "N2 Gas Pressure_Min" ("Tag Name")
        w398 = "O2 Gas Pressure _Value" ("Tag Name")
        w399 = "O2 Gas Pressure_Max" ("Tag Name")
        w406 = "O2 Gas Pressure_Min" ("Tag Name")
        n82 = call "Read Input Registers.vi"("error in (no error)"=w265, "quantity"=u16 25 ("Starting Address"), "starting address"=u16 0 ("Starting Address"), "MB session in"=w266) -> ("error out"=w261:errorcluster, "Registers"=w260:u16[], "MB session out"=w262:refnum<class "MB_Master.lvclass">)  [unwired: 5 in]
        n83 = Index Array(array=w260, index #1=21 ("index"), index #2=22 ("index"), index #3=23 ("index")) -> (element #1=w279:u16, element #2=w278:u16, element #3=w277:u16)
        n84 = Index Array(array=w260, index #1=3 ("index"), index #2=4 ("index"), index #3=5 ("index")) -> (element #1=w394:u16, element #2=w389:u16, element #3=w381:u16)
        n85 = Index Array(array=w260, index #1=18 ("index"), index #2=19 ("index"), index #3=20 ("index")) -> (element #1=w299:u16, element #2=w298:u16, element #3=w297:u16)
        n86 = Index Array(array=w260, index #1=6 ("index"), index #2=7 ("index"), index #3=8 ("index")) -> (element #1=w373:u16, element #2=w372:u16, element #3=w371:u16)
        n87 = Index Array(array=w260, index #1=9 ("index"), index #2=10 ("index"), index #3=11 ("index")) -> (element #1=w356:u16, element #2=w355:u16, element #3=w354:u16)
        n88 = Index Array(array=w260, index #1=12 ("index"), index #2=13 ("index"), index #3=14 ("index")) -> (element #1=w338:u16, element #2=w337:u16, element #3=w336:u16)
        n89 = Index Array(array=w260, index #1=0 ("index"), index #2=1 ("index"), index #3=2 ("index")) -> (element #1=w416:u16, element #2=w414:u16, element #3=w408:u16)
        n90 = Index Array(array=w260, index #1=15 ("index"), index #2=16 ("index"), index #3=17 ("index")) -> (element #1=w315:u16, element #2=w314:u16, element #3=w313:u16)
        n91 = call-poly <vilib>:"Write.vi"("error in (no error)"=w261, "Value"=w416, "Tag Name"=w406) -> ("error out"=w413:errorcluster)  [unwired: 8 in]
        n92 = call-poly <vilib>:"Read.vi"("error in (no error)"=w413, "Default"=u16 0, "Tag Name"=w406) -> ("error out"=w412:errorcluster, "Value"=→"Min_O2":u16)  [unwired: 7 in]
        n93 = call-poly <vilib>:"Read.vi"("Default"=u16 0, "Tag Name"=w392) -> ("error out"=w386:errorcluster, "Value"=→"Min_N2":u16)  [unwired: 8 in]
        n94 = call-poly <vilib>:"Write.vi"("error in (no error)"=w413, "Value"=w414, "Tag Name"=w399) -> ("error out"=w407:errorcluster)  [unwired: 8 in]
        n95 = call-poly <vilib>:"Read.vi"("error in (no error)"=w412, "Default"=u16 0, "Tag Name"=w399) -> ("error out"=w404:errorcluster, "Value"=→"Max_O2":u16)  [unwired: 7 in]
        n96 = call-poly <vilib>:"Read.vi"("Tag Name"=w329) -> ("error out"=w331:errorcluster, "Value"=→"Temp_Max":u16)  [unwired: 9 in]
        n97 = call-poly <vilib>:"Read.vi"("error in (no error)"=w386, "Default"=u16 0, "Tag Name"=w388) -> ("error out"=w379:errorcluster, "Value"=→"Max_N2":u16)  [unwired: 7 in]
        n98 = call-poly <vilib>:"Write.vi"("error in (no error)"=w407, "Value"=w408, "Tag Name"=w398) -> ()  [unwired: 8 in, 1 out]
        n99 = call-poly <vilib>:"Read.vi"("error in (no error)"=w331, "Tag Name"=w330) -> ("error out"=w308:errorcluster, "Value"=→"Temp_Min 2":u16)  [unwired: 8 in]
        n100 = call-poly <vilib>:"Read.vi"("error in (no error)"=w308, "Tag Name"=w312) -> ("error out"=w307:errorcluster, "Value"=→"Hum_Min":u16)  [unwired: 8 in]
        n101 = call-poly <vilib>:"Read.vi"("error in (no error)"=w307, "Tag Name"=w311) -> ("error out"=w318:errorcluster, "Value"=→"Hum_Max":u16)  [unwired: 8 in]
        n102 = call-poly <vilib>:"Read.vi"("error in (no error)"=w318, "Tag Name"=w310) -> ("error out"=w280:errorcluster, "Value"=→"Hum_Value":u16)  [unwired: 8 in]
        n103 = call-poly <vilib>:"Read.vi"("error in (no error)"=w280, "Default"=u16 0, "Tag Name"=w296) -> ("error out"=w303:errorcluster, "Value"=→"Spare AI-1_Min":u16)  [unwired: 7 in]
        n104 = call-poly <vilib>:"Read.vi"("error in (no error)"=w303, "Default"=u16 0, "Tag Name"=w294) -> ("error out"=w304:errorcluster, "Value"=→"Spare AI-1_Max":u16)  [unwired: 7 in]
        n105 = call-poly <vilib>:"Read.vi"("error in (no error)"=w304, "Default"=u16 0, "Tag Name"=w293) -> ("error out"=w272:errorcluster, "Value"=→"Spare AI-1_Value":u16)  [unwired: 7 in]
        n106 = call-poly <vilib>:"Read.vi"("error in (no error)"=w272, "Tag Name"=w274) -> ("error out"=w281:errorcluster, "Value"=→"Spare AI-2_Min":u16)  [unwired: 8 in]
        n107 = call-poly <vilib>:"Read.vi"("error in (no error)"=w281, "Tag Name"=w276) -> ("error out"=w282:errorcluster, "Value"=→"Spare AI-2_Max":u16)  [unwired: 8 in]
        n108 = call-poly <vilib>:"Read.vi"("error in (no error)"=w282, "Tag Name"=w275) -> ("error out"=w271:errorcluster, "Value"=→"Spare AI-2_Value":u16)  [unwired: 8 in]
        n109 = call-poly <vilib>:"Read.vi"("error in (no error)"=w379, "Default"=u16 0, "Tag Name"=w383) -> ("error out"=w367:errorcluster, "Value"=→"Value_N2":u16)  [unwired: 7 in]
        n110 = call-poly <vilib>:"Read.vi"("error in (no error)"=w367, "Tag Name"=w368) -> ("error out"=w366:errorcluster, "Value"=→"Vel_Min":u16)  [unwired: 8 in]
        n111 = call-poly <vilib>:"Read.vi"("error in (no error)"=w366, "Tag Name"=w365) -> ("error out"=w364:errorcluster, "Value"=→"Vel_Max":u16)  [unwired: 8 in]
        n112 = call-poly <vilib>:"Read.vi"("error in (no error)"=w364, "Tag Name"=w363) -> ("error out"=w350:errorcluster, "Value"=→"Vel_Value":u16)  [unwired: 8 in]
        n113 = call-poly <vilib>:"Read.vi"("error in (no error)"=w350, "Tag Name"=w349) -> ("error out"=w347:errorcluster, "Value"=→"N2 Gas Pressure 1_Min":u16)  [unwired: 8 in]
        n114 = call-poly <vilib>:"Read.vi"("error in (no error)"=w347, "Tag Name"=w348) -> ("error out"=w344:errorcluster, "Value"=→"N2 Gas Pressure 1_Max":u16)  [unwired: 8 in]
        n115 = call-poly <vilib>:"Read.vi"("error in (no error)"=w344, "Tag Name"=w343) -> ("error out"=w328:errorcluster, "Value"=→"N2 Gas Pressure 1_Value":u16)  [unwired: 8 in]
        n116 = call-poly <vilib>:"Read.vi"("error in (no error)"=w328, "Tag Name"=w327) -> ("Value"=→"Temp_Min":u16)  [unwired: 8 in, 1 out]
        n117 = call-poly <vilib>:"Read.vi"("error in (no error)"=w404, "Default"=u16 0, "Tag Name"=w398) -> ("error out"=w393:errorcluster, "Value"=→"Value_O2":u16)  [unwired: 7 in]
        n118 = call-poly <vilib>:"Write.vi"("error in (no error)"=w393, "Value"=w394, "Tag Name"=w392) -> ("error out"=w387:errorcluster)  [unwired: 8 in]
        n119 = call-poly <vilib>:"Write.vi"("error in (no error)"=w387, "Value"=w389, "Tag Name"=w388) -> ("error out"=w384:errorcluster)  [unwired: 8 in]
        n120 = call-poly <vilib>:"Write.vi"("error in (no error)"=w384, "Value"=w381, "Tag Name"=w383) -> ("error out"=w374:errorcluster)  [unwired: 8 in]
        n121 = call-poly <vilib>:"Write.vi"("error in (no error)"=w374, "Value"=w373, "Tag Name"=w368) -> ("error out"=w370:errorcluster)  [unwired: 8 in]
        n122 = call-poly <vilib>:"Write.vi"("error in (no error)"=w370, "Value"=w372, "Tag Name"=w365) -> ("error out"=w369:errorcluster)  [unwired: 8 in]
        n123 = call-poly <vilib>:"Write.vi"("error in (no error)"=w369, "Value"=w371, "Tag Name"=w363) -> ("error out"=w353:errorcluster)  [unwired: 8 in]
        n124 = call-poly <vilib>:"Write.vi"("error in (no error)"=w353, "Value"=w356, "Tag Name"=w349) -> ("error out"=w352:errorcluster)  [unwired: 8 in]
        n125 = call-poly <vilib>:"Write.vi"("error in (no error)"=w352, "Value"=w355, "Tag Name"=w348) -> ("error out"=w351:errorcluster)  [unwired: 8 in]
        n126 = call-poly <vilib>:"Write.vi"("error in (no error)"=w351, "Value"=w354, "Tag Name"=w343) -> ("error out"=w335:errorcluster)  [unwired: 8 in]
        n127 = call-poly <vilib>:"Write.vi"("error in (no error)"=w335, "Value"=w338, "Tag Name"=w327) -> ("error out"=w334:errorcluster)  [unwired: 8 in]
        n128 = call-poly <vilib>:"Write.vi"("error in (no error)"=w334, "Value"=w337, "Tag Name"=w329) -> ("error out"=w333:errorcluster)  [unwired: 8 in]
        n129 = call-poly <vilib>:"Write.vi"("error in (no error)"=w333, "Value"=w336, "Tag Name"=w330) -> ("error out"=w309:errorcluster)  [unwired: 8 in]
        n130 = call-poly <vilib>:"Write.vi"("error in (no error)"=w309, "Value"=w315, "Tag Name"=w312) -> ("error out"=w321:errorcluster)  [unwired: 8 in]
        n131 = call-poly <vilib>:"Write.vi"("error in (no error)"=w321, "Value"=w314, "Tag Name"=w311) -> ("error out"=w320:errorcluster)  [unwired: 8 in]
        n132 = call-poly <vilib>:"Write.vi"("error in (no error)"=w320, "Value"=w313, "Tag Name"=w310) -> ("error out"=w295:errorcluster)  [unwired: 8 in]
        n133 = call-poly <vilib>:"Write.vi"("error in (no error)"=w295, "Value"=w299, "Tag Name"=w296) -> ("error out"=w306:errorcluster)  [unwired: 8 in]
        n134 = call-poly <vilib>:"Write.vi"("error in (no error)"=w306, "Value"=w298, "Tag Name"=w294) -> ("error out"=w305:errorcluster)  [unwired: 8 in]
        n135 = call-poly <vilib>:"Write.vi"("error in (no error)"=w305, "Value"=w297, "Tag Name"=w293) -> ("error out"=w273:errorcluster)  [unwired: 8 in]
        n136 = call-poly <vilib>:"Write.vi"("error in (no error)"=w273, "Value"=w279, "Tag Name"=w274) -> ("error out"=w283:errorcluster)  [unwired: 8 in]
        n137 = call-poly <vilib>:"Write.vi"("error in (no error)"=w283, "Value"=w278, "Tag Name"=w276) -> ("error out"=w269:errorcluster)  [unwired: 8 in]
        n138 = call-poly <vilib>:"Write.vi"("error in (no error)"=w269, "Value"=w277, "Tag Name"=w275) -> ()  [unwired: 8 in, 1 out]
        n139 = Unbundle By Name(w271) -> ("status"=w401:bool)
        n140 = Or(x=w401, y="stop  3") -> (x .or. y?=w400:bool)
      }
      frame #3 {
        w431 = "Value_14" ("Tag Name")
        w432 = "Value_13" ("Tag Name")
        w446 = "Value_12" ("Tag Name")
        w447 = "Value_11" ("Tag Name")
        w448 = "Value_10" ("Tag Name")
        w449 = "Value_9" ("Tag Name")
        w466 = "Value_8" ("Tag Name")
        w471 = "Value_7" ("Tag Name")
        w476 = "Value_6" ("Tag Name")
        w483 = "Value_5" ("Tag Name")
        w489 = "Value_4" ("Tag Name")
        w495 = "Value_3" ("Tag Name")
        w498 = "Value_2" ("Tag Name")
        w508 = "Value_1" ("Tag Name")
        n141 = call-poly <vilib>:"Read.vi"("Tag Name"=w432) -> ("error out"=w430:errorcluster, "Value"=→"Value_13":bool)  [unwired: 9 in]
        n142 = call-poly <vilib>:"Read.vi"("error in (no error)"=w430, "Tag Name"=w431) -> ("error out"=w429:errorcluster, "Value"=→"Value_14":bool)  [unwired: 8 in]
        n143 = call "Read Discrete Inputs.vi"("error in (no error)"=w421, "quantity"=u16 14 ("Quantity"), "starting address"=u16 17 ("Starting Address"), "MB session in"=w424) -> ("error out"=w420:errorcluster, "Inputs"=w423:bool[], "MB session out"=w422:refnum<class "MB_Master.lvclass">)  [unwired: 5 in]
        n144 = Index Array(array=w423, index=2) -> (element=w493:bool)
        n145 = Index Array(array=w423, index=3) -> (element=w487:bool)
        n146 = Index Array(array=w423, index=4) -> (element=w484:bool)
        n147 = Index Array(array=w423, index=5) -> (element=w478:bool)
        n148 = Index Array(array=w423, index=6) -> (element=w472:bool)
        n149 = Index Array(array=w423, index=7) -> (element=w465:bool)
        n150 = Index Array(array=w423, index=0) -> (element=w509:bool)
        n151 = Index Array(array=w423, index=1) -> (element=w501:bool)
        n152 = Index Array(array=w423, index=8) -> (element=w453:bool)
        n153 = Index Array(array=w423, index=9) -> (element=w452:bool)
        n154 = Index Array(array=w423, index=10) -> (element=w451:bool)
        n155 = Index Array(array=w423, index=11) -> (element=w450:bool)
        n156 = Index Array(array=w423, index=12) -> (element=w436:bool)
        n157 = Index Array(array=w423, index=13) -> (element=w435:bool)
        n158 = call-poly <vilib>:"Write.vi"("error in (no error)"=w420, "Value"=w509, "Tag Name"=w508) -> ("error out"=w502:errorcluster)  [unwired: 8 in]
        n159 = call-poly <vilib>:"Write.vi"("error in (no error)"=w502, "Value"=w501, "Tag Name"=w498) -> ("error out"=w497:errorcluster)  [unwired: 8 in]
        n160 = call-poly <vilib>:"Write.vi"("error in (no error)"=w497, "Value"=w493, "Tag Name"=w495) -> ("error out"=w490:errorcluster)  [unwired: 8 in]
        n161 = call-poly <vilib>:"Write.vi"("error in (no error)"=w490, "Value"=w487, "Tag Name"=w489) -> ("error out"=w481:errorcluster)  [unwired: 8 in]
        n162 = call-poly <vilib>:"Write.vi"("error in (no error)"=w481, "Value"=w484, "Tag Name"=w483) -> ("error out"=w477:errorcluster)  [unwired: 8 in]
        n163 = call-poly <vilib>:"Write.vi"("error in (no error)"=w477, "Value"=w478, "Tag Name"=w476) -> ("error out"=w469:errorcluster)  [unwired: 8 in]
        n164 = call-poly <vilib>:"Write.vi"("error in (no error)"=w469, "Value"=w472, "Tag Name"=w471) -> ("error out"=w463:errorcluster)  [unwired: 8 in]
        n165 = call-poly <vilib>:"Write.vi"("error in (no error)"=w463, "Value"=w465, "Tag Name"=w466) -> ("error out"=w457:errorcluster)  [unwired: 8 in]
        n166 = call-poly <vilib>:"Write.vi"("error in (no error)"=w457, "Value"=w453, "Tag Name"=w449) -> ("error out"=w456:errorcluster)  [unwired: 8 in]
        n167 = call-poly <vilib>:"Write.vi"("error in (no error)"=w456, "Value"=w452, "Tag Name"=w448) -> ("error out"=w455:errorcluster)  [unwired: 8 in]
        n168 = call-poly <vilib>:"Write.vi"("error in (no error)"=w455, "Value"=w451, "Tag Name"=w447) -> ("error out"=w454:errorcluster)  [unwired: 8 in]
        n169 = call-poly <vilib>:"Write.vi"("error in (no error)"=w454, "Value"=w450, "Tag Name"=w446) -> ("error out"=w434:errorcluster)  [unwired: 8 in]
        n170 = call-poly <vilib>:"Write.vi"("error in (no error)"=w434, "Value"=w436, "Tag Name"=w432) -> ("error out"=w433:errorcluster)  [unwired: 8 in]
        n171 = call-poly <vilib>:"Write.vi"("error in (no error)"=w433, "Value"=w435, "Tag Name"=w431) -> ()  [unwired: 8 in, 1 out]
        n172 = call-poly <vilib>:"Read.vi"("error in (no error)"=w502, "Tag Name"=w508) -> ("error out"=w500:errorcluster, "Value"=→"Value_1":bool)  [unwired: 8 in]
        n173 = call-poly <vilib>:"Read.vi"("error in (no error)"=w500, "Tag Name"=w498) -> ("error out"=w496:errorcluster, "Value"=→"Value_2":bool)  [unwired: 8 in]
        n174 = call-poly <vilib>:"Read.vi"("error in (no error)"=w496, "Tag Name"=w495) -> ("error out"=w491:errorcluster, "Value"=→"Value_3":bool)  [unwired: 8 in]
        n175 = call-poly <vilib>:"Read.vi"("error in (no error)"=w491, "Tag Name"=w489) -> ("error out"=w482:errorcluster, "Value"=→"Value_4":bool)  [unwired: 8 in]
        n176 = call-poly <vilib>:"Read.vi"("error in (no error)"=w482, "Tag Name"=w483) -> ("error out"=w475:errorcluster, "Value"=→"Value_5":bool)  [unwired: 8 in]
        n177 = call-poly <vilib>:"Read.vi"("error in (no error)"=w475, "Tag Name"=w476) -> ("error out"=w470:errorcluster, "Value"=→"Value_6":bool)  [unwired: 8 in]
        n178 = call-poly <vilib>:"Read.vi"("error in (no error)"=w470, "Tag Name"=w471) -> ("error out"=w462:errorcluster, "Value"=→"Value_7":bool)  [unwired: 8 in]
        n179 = call-poly <vilib>:"Read.vi"("error in (no error)"=w462, "Tag Name"=w466) -> ("error out"=w445:errorcluster, "Value"=→"Value_8" →"Value_9":bool)  [unwired: 8 in]
        n180 = call-poly <vilib>:"Read.vi"("error in (no error)"=w445, "Tag Name"=w449) -> ("error out"=w444:errorcluster, "Value"=→"Value_10":bool)  [unwired: 8 in]
        n181 = call-poly <vilib>:"Read.vi"("error in (no error)"=w444, "Tag Name"=w448) -> ("error out"=w443:errorcluster)  [unwired: 8 in, 1 out]
        n182 = call-poly <vilib>:"Read.vi"("error in (no error)"=w443, "Tag Name"=w447) -> ("error out"=w442:errorcluster, "Value"=→"Value_11":bool)  [unwired: 8 in]
        n183 = call-poly <vilib>:"Read.vi"("error in (no error)"=w442, "Tag Name"=w446) -> ("Value"=→"Value_12":bool)  [unwired: 8 in, 1 out]
        n184 = Unbundle By Name(w429) -> ("status"=w505:bool)
        n185 = Or(x=w505, y="stop  4") -> (x .or. y?=w504:bool)
      }
      frame #4 {
        w522 = "RH_H2" ("Tag Name")
        w523 = "RH_H1" ("Tag Name")
        w524 = "RH_L2" ("Tag Name")
        w525 = "RH_L1" ("Tag Name")
        w539 = "Temp_H2" ("Tag Name")
        w540 = "Temp_H1" ("Tag Name")
        w541 = "Temp_L2" ("Tag Name")
        w547 = "Temp_L1" ("Tag Name")
        w552 = "N22_H2" ("Tag Name")
        w553 = "N22_H1" ("Tag Name")
        w554 = "N22_L2" ("Tag Name")
        w555 = "N22_L1" ("Tag Name")
        w571 = "Vel_H2" ("Tag Name")
        w572 = "Vel_H1" ("Tag Name")
        w573 = "Vel_L2" ("Tag Name")
        w574 = "Vel_L1" ("Tag Name")
        w583 = "N21_H2" ("Tag Name")
        w584 = "N21_H1" ("Tag Name")
        w585 = "N21_L2" ("Tag Name")
        w586 = "N21_L1" ("Tag Name")
        w640 = "O2_H2" ("Tag Name")
        w643 = "O2_H1" ("Tag Name")
        w635 = "O2_L2" ("Tag Name")
        w651 = "O2_L1" ("Tag Name")
        n186 = call-poly <vilib>:"Read.vi"("Tag Name"=w651) -> ("error out"=w649:errorcluster, "Value"=→"Min_O2 2":u16)  [unwired: 9 in]
        n187 = call-poly <vilib>:"Read.vi"("error in (no error)"=w649, "Tag Name"=w635) -> ("error out"=w642:errorcluster, "Value"=→"Max_O2 2":u16)  [unwired: 8 in]
        n188 = call "Read Input Registers.vi"("error in (no error)"=w517, "quantity"=u16 24 ("Quantity"), "starting address"=u16 100 ("Starting Address"), "MB session in"=w513) -> ("error out"=w516:errorcluster, "Registers"=w514:u16[], "MB session out"=w515:refnum<class "MB_Master.lvclass">)  [unwired: 5 in]
        n189 = Index Array(array=w514, index #1=0 ("index"), index #2=1 ("index"), index #3=2 ("index"), index #4=3 ("index")) -> (element #1=w655:u16, element #2=w654:u16, element #3=w653:u16, element #4=w652:u16)
        n190 = Index Array(array=w514, index #1=8 ("index"), index #2=9 ("index"), index #3=10 ("index"), index #4=11 ("index")) -> (element #1=w622:u16, element #2=w621:u16, element #3=w620:u16, element #4=w619:u16)
        n191 = Index Array(array=w514, index #1=12 ("index"), index #2=13 ("index"), index #3=14 ("index"), index #4=15 ("index")) -> (element #1=w614:u16, element #2=w613:u16, element #3=w612:u16, element #4=w611:u16)
        n192 = Index Array(array=w514, index #1=16 ("index"), index #2=17 ("index"), index #3=18 ("index"), index #4=19 ("index")) -> (element #1=w606:u16, element #2=w605:u16, element #3=w604:u16, element #4=w603:u16)
        n193 = Index Array(array=w514, index #1=4 ("index"), index #2=5 ("index"), index #3=6 ("index"), index #4=7 ("index")) -> (element #1=w630:u16, element #2=w629:u16, element #3=w628:u16, element #4=w627:u16)
        n194 = Index Array(array=w514, index #1=20 ("index"), index #2=21 ("index"), index #3=22 ("index"), index #4=23 ("index")) -> (element #1=w598:u16, element #2=w597:u16, element #3=w596:u16, element #4=w595:u16)
        n195 = call-poly <vilib>:"Write.vi"("error in (no error)"=w516, "Value"=w655, "Tag Name"=w651) -> ("error out"=w650:errorcluster)  [unwired: 8 in]
        n196 = call-poly <vilib>:"Write.vi"("Value"=w622, "Tag Name"=w574) -> ("error out"=w577:errorcluster)  [unwired: 9 in]
        n197 = call-poly <vilib>:"Write.vi"("error in (no error)"=w650, "Value"=w654, "Tag Name"=w635) -> ("error out"=w648:errorcluster)  [unwired: 8 in]
        n198 = call-poly <vilib>:"Write.vi"("error in (no error)"=w577, "Value"=w621, "Tag Name"=w573) -> ("error out"=w576:errorcluster)  [unwired: 8 in]
        n199 = call-poly <vilib>:"Write.vi"("error in (no error)"=w648, "Value"=w653, "Tag Name"=w643) -> ("error out"=w647:errorcluster)  [unwired: 8 in]
        n200 = call-poly <vilib>:"Read.vi"("error in (no error)"=w642, "Tag Name"=w643) -> ("error out"=w641:errorcluster, "Value"=→"Value_O2 2":u16)  [unwired: 8 in]
        n201 = call-poly <vilib>:"Read.vi"("Tag Name"=w541) -> ("Value"=→"Temp_Max 2":u16)  [unwired: 9 in, 1 out]
        n202 = call-poly <vilib>:"Write.vi"("error in (no error)"=w576, "Value"=w620, "Tag Name"=w572) -> ("error out"=w575:errorcluster)  [unwired: 8 in]
        n203 = call-poly <vilib>:"Write.vi"("error in (no error)"=w647, "Value"=w652, "Tag Name"=w640) -> ("error out"=w594:errorcluster)  [unwired: 8 in]
        n204 = call-poly <vilib>:"Write.vi"("error in (no error)"=w594, "Value"=w630, "Tag Name"=w586) -> ("error out"=w593:errorcluster)  [unwired: 8 in]
        n205 = call-poly <vilib>:"Write.vi"("error in (no error)"=w593, "Value"=w629, "Tag Name"=w585) -> ("error out"=w592:errorcluster)  [unwired: 8 in]
        n206 = call-poly <vilib>:"Write.vi"("error in (no error)"=w592, "Value"=w628, "Tag Name"=w584) -> ("error out"=w591:errorcluster)  [unwired: 8 in]
        n207 = call-poly <vilib>:"Read.vi"("error in (no error)"=w641, "Tag Name"=w640) -> ("error out"=w590:errorcluster, "Value"=→"Value_O2 3":u16)  [unwired: 8 in]
        n208 = call-poly <vilib>:"Read.vi"("error in (no error)"=w590, "Tag Name"=w586) -> ("error out"=w589:errorcluster, "Value"=→"Min_N2 2":u16)  [unwired: 8 in]
        n209 = call-poly <vilib>:"Read.vi"("error in (no error)"=w589, "Tag Name"=w585) -> ("error out"=w588:errorcluster, "Value"=→"Max_N2 2":u16)  [unwired: 8 in]
        n210 = call-poly <vilib>:"Read.vi"("Tag Name"=w540) -> ("Value"=→"Temp_Min 3":u16)  [unwired: 9 in, 1 out]
        n211 = call-poly <vilib>:"Read.vi"("error in (no error)"=w588, "Tag Name"=w584) -> ("error out"=w587:errorcluster, "Value"=→"Value_N2 2":u16)  [unwired: 8 in]
        n212 = call-poly <vilib>:"Write.vi"("error in (no error)"=w575, "Value"=w619, "Tag Name"=w571) -> ("error out"=w556:errorcluster)  [unwired: 8 in]
        n213 = call-poly <vilib>:"Write.vi"("error in (no error)"=w556, "Value"=w614, "Tag Name"=w555) -> ("error out"=w559:errorcluster)  [unwired: 8 in]
        n214 = call-poly <vilib>:"Write.vi"("error in (no error)"=w559, "Value"=w613, "Tag Name"=w554) -> ("error out"=w558:errorcluster)  [unwired: 8 in]
        n215 = call-poly <vilib>:"Write.vi"("error in (no error)"=w558, "Value"=w612, "Tag Name"=w553) -> ("error out"=w557:errorcluster)  [unwired: 8 in]
        n216 = call-poly <vilib>:"Write.vi"("error in (no error)"=w557, "Value"=w611, "Tag Name"=w552) -> ("error out"=w543:errorcluster)  [unwired: 8 in]
        n217 = call-poly <vilib>:"Write.vi"("error in (no error)"=w543, "Value"=w606, "Tag Name"=w547) -> ("error out"=w546:errorcluster)  [unwired: 8 in]
        n218 = call-poly <vilib>:"Write.vi"("error in (no error)"=w546, "Value"=w605, "Tag Name"=w541) -> ("error out"=w545:errorcluster)  [unwired: 8 in]
        n219 = call-poly <vilib>:"Write.vi"("error in (no error)"=w545, "Value"=w604, "Tag Name"=w540) -> ("error out"=w544:errorcluster)  [unwired: 8 in]
        n220 = call-poly <vilib>:"Write.vi"("error in (no error)"=w544, "Value"=w603, "Tag Name"=w539) -> ("error out"=w534:errorcluster)  [unwired: 8 in]
        n221 = call-poly <vilib>:"Write.vi"("error in (no error)"=w534, "Value"=w598, "Tag Name"=w525) -> ("error out"=w533:errorcluster)  [unwired: 8 in]
        n222 = call-poly <vilib>:"Write.vi"("error in (no error)"=w533, "Value"=w597, "Tag Name"=w524) -> ("error out"=w532:errorcluster)  [unwired: 8 in]
        n223 = call-poly <vilib>:"Write.vi"("error in (no error)"=w532, "Value"=w596, "Tag Name"=w523) -> ("error out"=w531:errorcluster)  [unwired: 8 in]
        n224 = call-poly <vilib>:"Write.vi"("error in (no error)"=w591, "Value"=w627, "Tag Name"=w583) -> ()  [unwired: 8 in, 1 out]
        n225 = call-poly <vilib>:"Write.vi"("error in (no error)"=w531, "Value"=w595, "Tag Name"=w522) -> ()  [unwired: 8 in, 1 out]
        n226 = call-poly <vilib>:"Read.vi"("Tag Name"=w539) -> ("error out"=w530:errorcluster, "Value"=→"Temp_Min 4":u16)  [unwired: 9 in]
        n227 = call-poly <vilib>:"Read.vi"("error in (no error)"=w530, "Tag Name"=w525) -> ("error out"=w529:errorcluster, "Value"=→"Hum_Min 2":u16)  [unwired: 8 in]
        n228 = call-poly <vilib>:"Read.vi"("error in (no error)"=w529, "Tag Name"=w524) -> ("error out"=w528:errorcluster, "Value"=→"Hum_Max 2":u16)  [unwired: 8 in]
        n229 = call-poly <vilib>:"Read.vi"("error in (no error)"=w528, "Tag Name"=w523) -> ("error out"=w527:errorcluster, "Value"=→"Hum_Value  2":u16)  [unwired: 8 in]
        n230 = call-poly <vilib>:"Read.vi"("error in (no error)"=w587, "Tag Name"=w583) -> ("error out"=w578:errorcluster, "Value"=→"Value_N2 3":u16)  [unwired: 8 in]
        n231 = call-poly <vilib>:"Read.vi"("error in (no error)"=w578, "Tag Name"=w574) -> ("error out"=w569:errorcluster, "Value"=→"Vel_Min 2":u16)  [unwired: 8 in]
        n232 = call-poly <vilib>:"Read.vi"("error in (no error)"=w569, "Tag Name"=w573) -> ("error out"=w568:errorcluster, "Value"=→"Vel_Max 2":u16)  [unwired: 8 in]
        n233 = call-poly <vilib>:"Read.vi"("error in (no error)"=w568, "Tag Name"=w572) -> ("error out"=w567:errorcluster, "Value"=→"Vel_Value 2":u16)  [unwired: 8 in]
        n234 = call-poly <vilib>:"Read.vi"("error in (no error)"=w567, "Tag Name"=w571) -> ("error out"=w563:errorcluster, "Value"=→"Vel_Value 3":u16)  [unwired: 8 in]
        n235 = call-poly <vilib>:"Read.vi"("error in (no error)"=w563, "Tag Name"=w555) -> ("error out"=w562:errorcluster, "Value"=→"N2 Gas Pressure 1_Min 2":u16)  [unwired: 8 in]
        n236 = call-poly <vilib>:"Read.vi"("error in (no error)"=w562, "Tag Name"=w554) -> ("error out"=w561:errorcluster, "Value"=→"N2 Gas Pressure 1_Max 2":u16)  [unwired: 8 in]
        n237 = call-poly <vilib>:"Read.vi"("error in (no error)"=w561, "Tag Name"=w553) -> ("error out"=w560:errorcluster, "Value"=→"N2 Gas Pressure 1_Value 2":u16)  [unwired: 8 in]
        n238 = call-poly <vilib>:"Read.vi"("error in (no error)"=w560, "Tag Name"=w552) -> ("error out"=w542:errorcluster, "Value"=→"N2 Gas Pressure 1_Value 3":u16)  [unwired: 8 in]
        n239 = call-poly <vilib>:"Read.vi"("error in (no error)"=w542, "Tag Name"=w547) -> ("Value"=→"Temp_Min 5":u16)  [unwired: 8 in, 1 out]
        n240 = call-poly <vilib>:"Read.vi"("error in (no error)"=w527, "Tag Name"=w522) -> ("error out"=w526:errorcluster, "Value"=→"Hum_Value  3":u16)  [unwired: 8 in]
        n241 = Unbundle By Name(w526) -> ("status"=w637:bool)
        n242 = Or(x="stop  5", y=w637) -> (x .or. y?=w636:bool)
      }
    }
  }
  n243 = call-dynamic "Close Session.vi"("error in (no error)"=w6, "MB session in"=w7) -> ("error out"=→"error out":errorcluster)  [unwired: 9 in]
